vi "updateFilePath.vi"(8 "error in (no error)":errorcluster, 10 "path":string, 11 "playFileAction in":refnum<class "playFileAction.lvclass">) -> (0 "error out":errorcluster, 2 "timeLength":dbl, 3 "playFileAction out":refnum<class "playFileAction.lvclass">)   [LabVIEW 2011, in "Views.lvlib" / "ScriptEditor.lvlib" / "playFileAction.lvclass"]
uses:
  playFileAction.lvclass
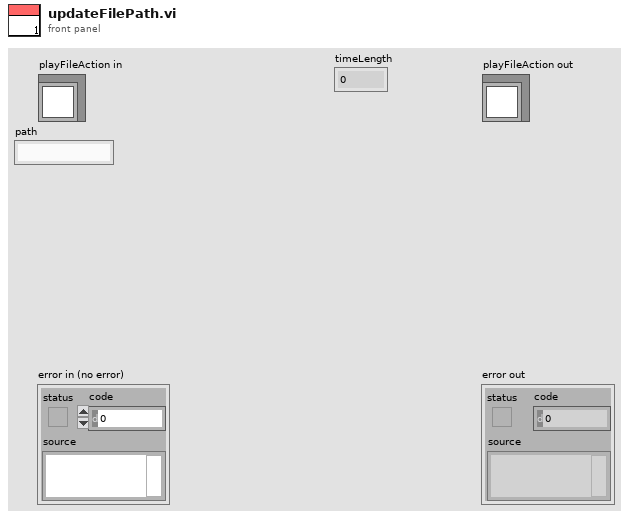
[diagram p1: front panel]
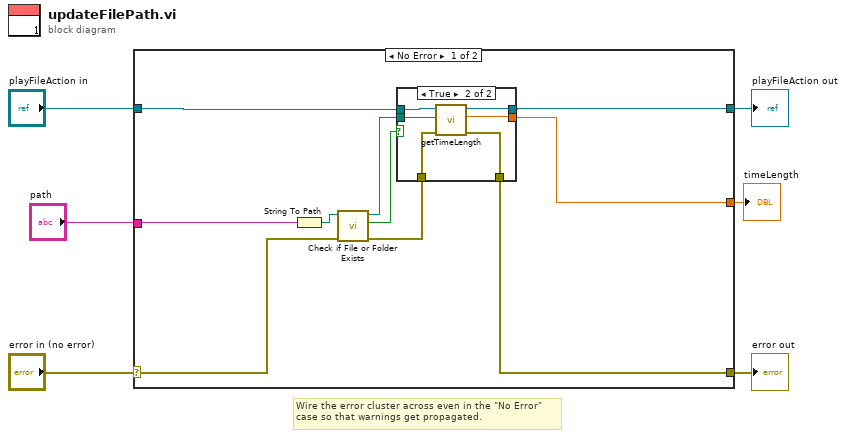
[diagram p0: block diagram]
diagram:
  # "Wire the error cluster across even in the \"No Error\"\ncase so that warnings get propagated."
  n1 = case shown="No Error" "error in (no error)" {
    selector: "error in (no error)" -> [w8 w26]
    tunnel: [w9 w26] -> w5
    tunnel: [w11 w25] -> w3
    tunnel: "playFileAction in" -> [w12 w25]
    tunnel: [w10 _] -> w2
    tunnel: "path" -> [w7 _]
    frame No Error {
      n2 = String To Path(string=w7) -> (path=w13:path)
      n3 = call <vilib>:"Check if File or Folder Exists.vi"("error in (no error)"=w8, "path"=w13) -> ("error out"=w16:errorcluster, "file or folder exists?"=w14:bool, "dup path"=w15:path)  [unwired: 7 in]
      n4 = case shown="True" w14 {
        tunnel: w12 -> [w18 w24]
        tunnel: [w18 w23] -> w11
        tunnel: [w17 w22] -> w9
        tunnel: w16 -> [w17 w21]
        tunnel: w15 -> [_ w20]
        tunnel: [_ w19] -> w10
        frame False {
        }
        frame True {
          n5 = call "getTimeLength.vi"("error in (no error)"=w21, "Path"=w20, "playFileAction"=w24) -> ("error out"=w22:errorcluster, "timeLength"=w19:dbl, "playFileAction out"=w23:refnum<class "playFileAction.lvclass">)  [unwired: 6 in]
        }
      }
    }
    frame Error {
    }
  }
  "error out" <- w5
  "playFileAction out" <- w3
  "timeLength" <- w2
